vi "PM Read Test.vi"() -> ()   [LabVIEW 2018]
panel:
  out "Power":dbl
  in  "stop":bool
  in  "Average Count":i32=10 min=1 step=1
  in  "Wavelength [nm]":dbl=1300.0 caption="Wavelength (0.0)"
  in  "Avg. Time (0.0) [sec.]":dbl=0.1 caption="Average Time (0.0)" min=0.1 max=5.0 step=0.1
  out "Average Count 2":i32 caption="Average Time"
  out "Avg. Time  [sec.]":dbl caption="Average Time"
  out "Wavelength [nm] 2":dbl caption="Wavelength"
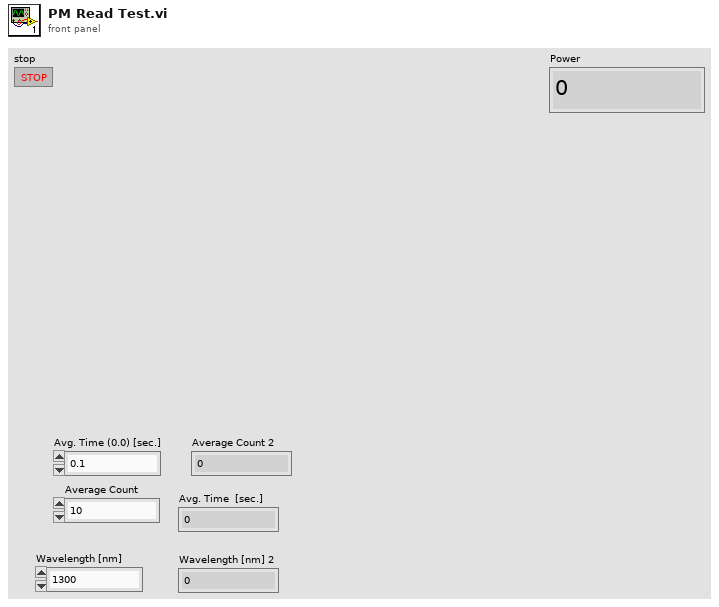
[diagram p1: front panel]
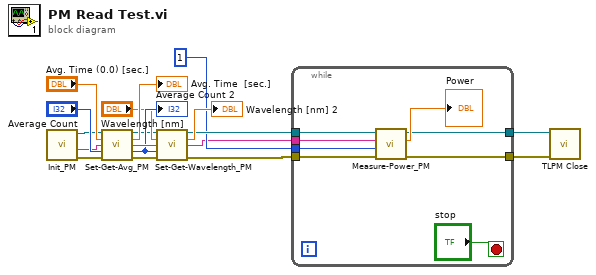
[diagram p0: block diagram]
diagram:
  n1 = call "Init_PM.vi"() -> ("error out"=w8:errorcluster, "Sensor Name"=w9:string, "instrument handle out"=w10:refnum<visa-resource-name>)  [unwired: 9 in]
  n2 = call "Set-Get-Avg_PM.vi"("instrument handle"=w10, "Average Time (0.0)"="Avg. Time (0.0) [sec.]", "Sensor"=w9, "Average Count"="Average Count", "error in (no error)"=w8) -> ("instrument handle out"=w6:refnum<visa-resource-name>, "Average Time"=→"Avg. Time  [sec.]":dbl, "Sensor 2"=w15:string, "Average Count"=w14:i32, "error out"=w17:errorcluster)  [unwired: 6 in]
  "Average Count 2" <- w14
  n3 = call "Set-Get-Wavelength_PM.vi"("instrument handle"=w6, "Wavelength"="Wavelength [nm]", "Sensor Name"=w15, "Average Count"=w14, "error in (no error)"=w17) -> ("instrument handle out"=w5:refnum<visa-resource-name>, "Wavelength"=→"Wavelength [nm] 2":dbl, "Sensor Name 2"=w3:string, "error out"=w7:errorcluster)  [unwired: 6 in, 1 out]
  n4 = while {
    tunnel: w7 -> [w26]
    tunnel: w5 -> [w25]
    tunnel: 1 ("Numeric") -> [w24]
    tunnel: w3 -> [w23]
    tunnel: [w20] -> w2
    tunnel: [w19] -> w1
    stop <- "stop" stop-if-true
    n5 = call "Measure-Power_PM.vi"("error in (no error)"=w26, "Numeric"=w24, "Sensor"=w23, "instrument handle"=w25) -> ("error out"=w20:errorcluster, "Power"=→"Power":dbl, "instrument handle out"=w19:refnum<visa-resource-name>)  [unwired: 5 in]
  }
  n6 = call "TLPM Close.vi"("error in (no error)"=w2, "instrument handle"=w1) -> ()  [unwired: 9 in, 1 out]
